vi "PressureCalibration(SubVI).vi"() -> ()   [LabVIEW 2013, in "Medimatic.lvlib"]
uses:
  Medimatic.lvlib
  Globals/DataAcqRecordPathGlobal.vi
  Controls/Enum Save Action Events.ctl
panel:
  in  "Cancel":bool
  in  "CurrentPressure":dbl
  in  "SavePresBtn":bool
  # "Pressure Calibration"
  # "Please type in the current pressure"
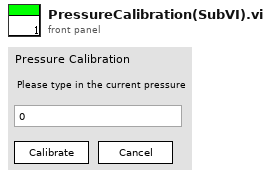
[diagram p1: front panel]
types:
  T1 = enum16{"Set", "Init", "Get Pressure", "Set Pressure", "Get"}
  T2 = typedef "Medimatic.lvlib/Enum Save Action Events.ctl" = enum16{"LoadReportPath", "SaveReportPath", "LoadDataPath", "SaveDataPath", "Load PressureFactor", "Save PressureFactor", "Init", "Load Listbox", "Save Listbox", "LoadHospInfo", "SaveHospInfo"}
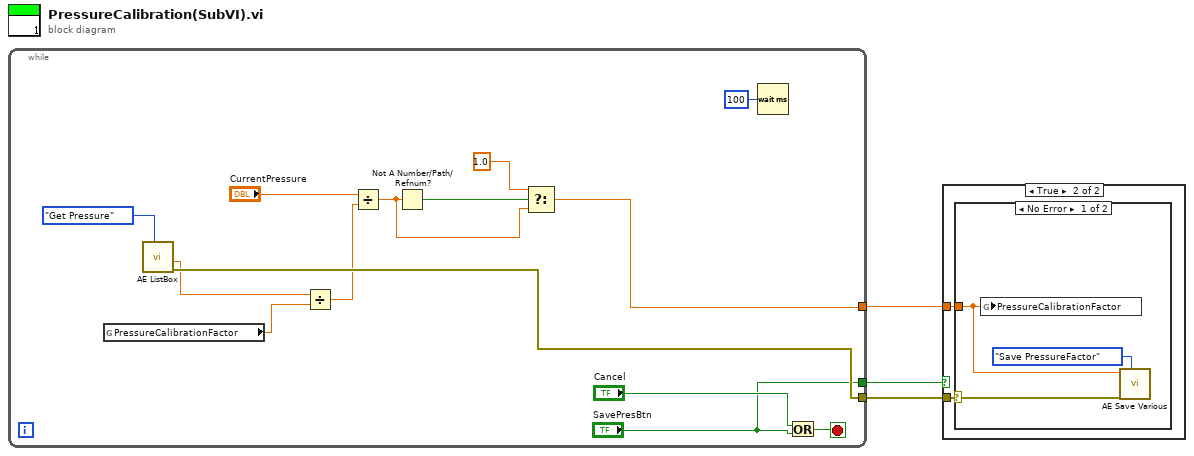
[diagram p0: block diagram]
diagram:
  n1 = while {
    tunnel: [w16] -> w3
    tunnel: [w6] -> w2
    tunnel: ["SavePresBtn"] -> w1
    stop <- w11 stop-if-true
    n2 = global read "DataAcqRecordPathGlobal.vi" "PressureCalibrationFactor"() -> (w15:dbl)
    n3 = call "AE ListBox.vi"("Action"=T1."Get Pressure") -> ("error out"=w16:errorcluster, "output pressure"=w13:dbl)  [unwired: 8 in, 1 out]
    n4 = Divide(x=w13, y=w15) -> (x/y=w14:dbl)
    n5 = Divide(x="CurrentPressure", y=w14) -> (x/y=w5:dbl)
    n6 = Not A Number/Path/Refnum?(number/path/refnum=w5) -> (NaN/Path/Refnum?=w7:bool)
    n7 = Select(t=1.0, s=w7, f=w5) -> (s? t:f=w6:dbl)
    n8 = Wait (ms)(milliseconds to wait=u32 100) -> ()  [unwired: 1 out]
    n9 = Or(x="Cancel", y="SavePresBtn") -> (x .or. y?=w11:bool)
  }
  n10 = case shown="True" w1 {
    tunnel: w3 -> [_ w19]
    tunnel: w2 -> [_ w18]
    frame False {
    }
    frame True {
      n11 = case shown="No Error" w19 {
        selector: w19 -> [w22 _]
        tunnel: w18 -> [w20 _]
        frame No Error {
          n12 = global write "DataAcqRecordPathGlobal.vi" "PressureCalibrationFactor"(w20) -> ()
          n13 = call "AE Save Various.vi"("error in (no error)"=w22, "Variant In"=w20, "Action"=Enum_Save_Action_Events."Save PressureFactor") -> ()  [unwired: 6 in, 2 out]
        }
        frame Error {
        }
      }
    }
  }
